vi "AVS_UseHighResADC.vi"(1 "a_Enable":u8, 2 "a_hDevice":i32) -> (0 "Output Value":i32)   [LabVIEW 2020]
uses:
  AvaSpecX64-DLL_9.4/avaspecx64.dll
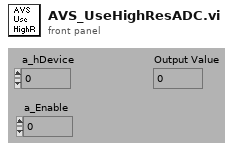
[diagram p1: front panel]
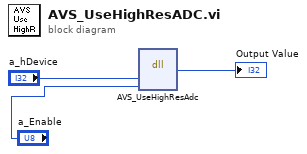
[diagram p0: block diagram]
diagram:
  n1 = dll-call lib="C:/AvaSpecX64-DLL_9.4/avaspecx64.dll" fn="AVS_UseHighResAdc"("a_hDevice"="a_hDevice", "a_Enable"="a_Enable") -> ("return type"=→"Output Value":i32)  [unwired: 5 in, 2 out]
